vi "CreateConstants.vi"(7 "PythonConverter_BD in":refnum<class "PyConvBD.lvclass">, 8 "error in":errorcluster, 11 "Diagram in":refnum<class "Diagram.lvclass">) -> (0 "error out":errorcluster, 3 "Diagram out":refnum<class "Diagram.lvclass">, 4 "create constants":string, 5 "PythonConverter_BD out":refnum<class "PyConvBD.lvclass">)   [LabVIEW 2014, in "Raspberry Pi Compatible Compiler for LabVIEW.lvlib" / "Diagram.lvclass"]
uses:
  Diagram.lvclass
  Python/PythonConverter_BD/PyConvBD.lvclass
  Diagram.lvclass/Diagram.ctl
  Python/Parsing/ClassTypeTD.ctl
  Constant/Constant.lvclass
  Python/Parsing/Python Functions.lvlib
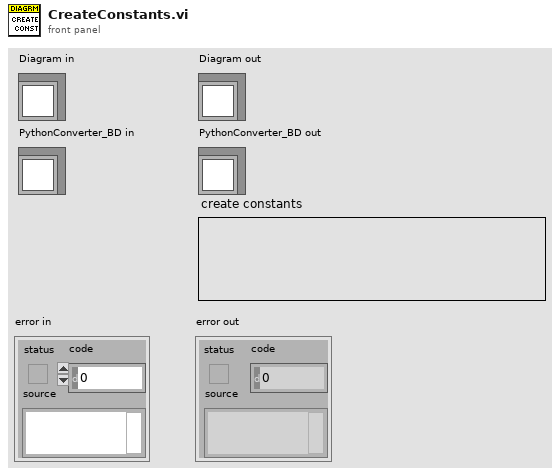
[diagram p1: front panel]
types:
  T1 = typedef "Raspberry Pi Compatible Compiler for LabVIEW.lvlib/Python Functions.lvlib/ClassTypeTD.ctl" = enum16{"class", "function"}
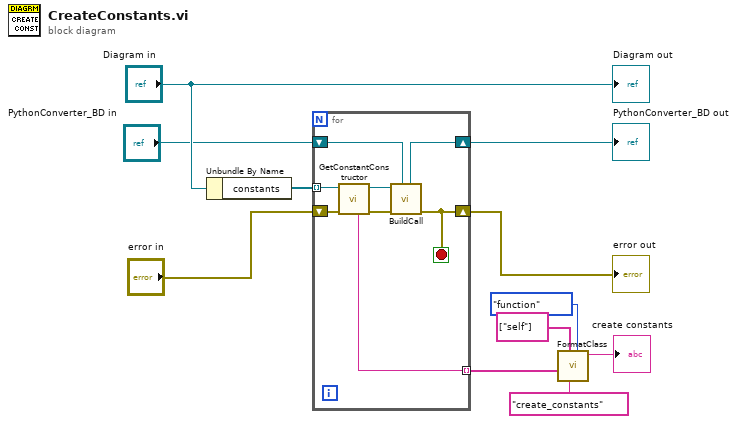
[diagram p0: block diagram]
diagram:
  n1 = Unbundle By Name("Diagram in") -> ("constants"=w11:refnum<class "Constant.lvclass">[])
  n2 = for {
    tunnel: w11 -> [w19] mode=indexing
    shift-right: [w12] -> w8
    shift-left: "error in" -> [w18]
    tunnel: [w17] -> w2 mode=indexing
    shift-right: [w13] -> w6
    shift-left: "PythonConverter_BD in" -> [w14]
    stop <- w12 stop-if-true
    n3 = call "GetConstantConstructor.vi"("error in"=w18, "Constant in"=w19) -> ("error out"=w16:errorcluster, "Constant out"=w15:refnum<class "Constant.lvclass">, "constant"=w17:string)  [unwired: 5 in]
    n4 = call "BuildCall.vi"("PythonConverter_BD in"=w14, "error in"=w16, "Constant in"=w15) -> ("error out"=w12:errorcluster, "PythonConverter_BD out"=w13:refnum<class "PyConvBD.lvclass">)  [unwired: 6 in, 1 out]
  }
  "error out" <- w8
  "PythonConverter_BD out" <- w6
  n5 = call "FormatClass.vi"("type"=ClassTypeTD."function", "name"="create_constants" ("initial string"), "parameters/ancestors"=string[] ["self"], "body"=w2) -> ("python"=→"create constants":string)  [unwired: 7 in]
  "Diagram out" <- "Diagram in"
